vi "ReplceColor.vi"(11 "Color Box":u32(colorbox)=16711680) -> (3 "Array":u32[][](array[numeric]))   [LabVIEW 2017]
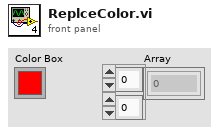
[diagram p1: front panel]
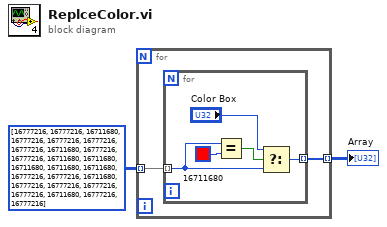
[diagram p0: block diagram]
diagram:
  n1 = for {
    tunnel: u32[][] [[16777216, 16777216, 16711680, 16777216, 16777216], [16777216, 16777216, 16711680, 16777216, 16777216], [16711680, 16711680, 16711680, 16711680, 16711680], [16777216, 16777216, 16711680, 16777216, 16777216], [16777216, 16777216, 16711680, 16777216, 16777216]] ("Bitmap") -> [w4] mode=indexing
    tunnel: [w3] -> w2 mode=indexing
    n2 = for {
      tunnel: w4 -> [w7] mode=indexing
      tunnel: [w6] -> w3 mode=indexing
      n3 = Equal?(x=w7, y=u32 16711680) -> (x = y?=w8:bool)
      n4 = Select(t="Color Box", s=w8, f=w7) -> (s? t:f=w6:u32)
    }
  }
  "Array" <- w2
